vi "LoadDynamicDependency.vi"(7 "SMO in":refnum<class "SMO.lvclass">, 8 "error in (no error)":errorcluster, 10 "HAL Folder (Subsystems)":string="Subsystems", 11 "Camera":string) -> (0 "error out":errorcluster, 3 "SMO out":refnum<class "SMO.lvclass">)   [LabVIEW 2013, in "Microscope.lvclass"]
uses:
  Subsystems/Microscope/Microscope.lvclass
  <vilib>/JKI/JKI SMO/SMO/SMO.lvclass
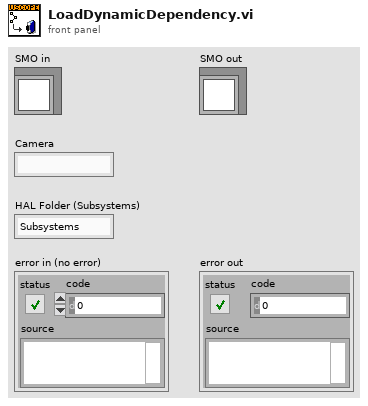
[diagram p1: front panel]
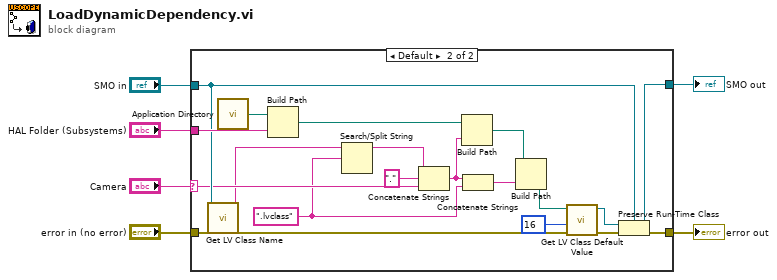
[diagram p0: block diagram]
diagram:
  n1 = case shown="Default" "Camera" {
    selector: "Camera" -> [_ w16]
    tunnel: "SMO in" -> [w8 w20]
    tunnel: "error in (no error)" -> [w7 w18]
    tunnel: [w7 w22] -> w3
    tunnel: [w8 w10] -> w5
    tunnel: "HAL Folder (Subsystems)" -> [_ w21]
    frame "" {
    }
    frame Default {
      w13 = ".lvclass" ("search string/char (-)")
      n2 = call <vilib>:"Get LV Class Name.vi"("error in (no error)"=w18, "object"=w20) -> ("error out"=w17:errorcluster, "class name"=w12:string)  [unwired: 8 in]
      n3 = call <vilib>:"Application Directory.vi"() -> ("Application Directory"=w27:path)
      n4 = Build Path(base path=w27, name or relative path=w21) -> (appended path=w26:path)
      n5 = Search/Split String(string=w12, search string/char (-)=w13) -> (substring before match=w19:string)  [unwired: 1 in, 2 out]
      n6 = Concatenate Strings(w19, "." ("string"), w16) -> (w14:string)
      n7 = Build Path(base path=w26, name or relative path=w14) -> (appended path=w11:path)
      n8 = Concatenate Strings(w14, w13) -> (w15:string)
      n9 = Build Path(base path=w11, name or relative path=w15) -> (appended path=w9:path)
      n10 = call <vilib>:"Get LV Class Default Value.vi"("error in (no error)"=w17, "options"=u32 16, "class path"=w9) -> ("error out"=w24:errorcluster, "object"=w25:refnum<class>)  [unwired: 7 in]
      n11 = Preserve Run-Time Class(object in=w25, error in=w24, 2:w20) -> (object out=w10:refnum<class "SMO.lvclass">, error out=w22:errorcluster)
    }
  }
  "SMO out" <- w5
  "error out" <- w3
